vi "Get spec limits.vi"(0 "Zaber":T1={"Serial port handle"="", "Axis"="", "Controller #"=0, "Min position"=0.0, "Max position"=0.0, "Min velocity"=0.0, "Max velocity"=0.0, "Firmware"="", "Device ID"=0, "Variable event"=refnum, "Variable ref"=refnum, "Resolution, usteps/step"=0, "Serial port semaphore"=refnum, "Joystick buttons"={"MinDir"=1, "MaxDir"=2, "MedSpeed"=5, "HighSpeed"=6}} {"Joystick buttons"."HighSpeed" min=1 max=25 step=1; "Joystick buttons"."MedSpeed" min=1 max=25 step=1; "Joystick buttons"."MaxDir" min=1 max=25 step=1; "Joystick buttons"."MinDir" min=1 max=25 step=1}, 5 "error in":errorcluster) -> (14 "Zaber out":T1={"Serial port handle"="", "Axis"="", "Controller #"=0, "Min position"=0.0, "Max position"=0.0, "Min velocity"=0.0, "Max velocity"=0.0, "Firmware"="", "Device ID"=0, "Variable event"=refnum, "Variable ref"=refnum, "Resolution, usteps/step"=0, "Serial port semaphore"=refnum, "Joystick buttons"={"MinDir"=1, "MaxDir"=2, "MedSpeed"=5, "HighSpeed"=6}} {"Joystick buttons"."HighSpeed" min=1 max=25 step=1; "Joystick buttons"."MedSpeed" min=1 max=25 step=1; "Joystick buttons"."MaxDir" min=1 max=25 step=1; "Joystick buttons"."MinDir" min=1 max=25 step=1}, 15 "MAX velocity, mm/s":dbl, 16 "MIN velociry, mm/s":dbl, 17 "MIN position, mm":dbl, 19 "error out":errorcluster)   [LabVIEW 2018]
uses:
  Zaber.ctl
  GenericDataEvent/GenericEvent.ctl
  ZaberVariables.ctl
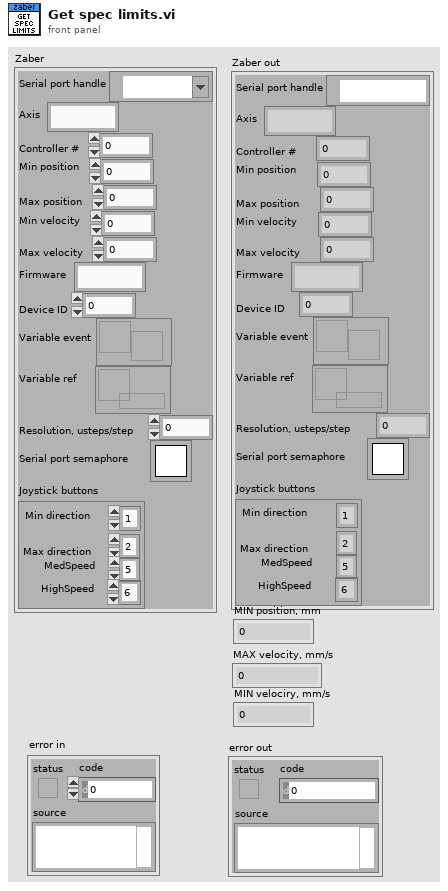
[diagram p1: front panel]
types:
  T1 = typedef "Zaber.ctl" = cluster{"Serial port handle":refnum<visa-resource-name>, "Axis":string, "Controller #":u8, "Min position":dbl, "Max position":dbl, "Min velocity":dbl, "Max velocity":dbl, "Firmware":string, "Device ID":i32, "Variable event":T2, "Variable ref":refnum<data-value>, "Resolution, usteps/step":i32, "Serial port semaphore":T3, "Joystick buttons":cluster{"MinDir":i32, "MaxDir":i32, "MedSpeed":i32, "HighSpeed":i32}}
  T2 = typedef "GenericEvent.ctl" = refnum<user-event>
  T3 = typedef "Semaphore RefNum" = refnum<k1>
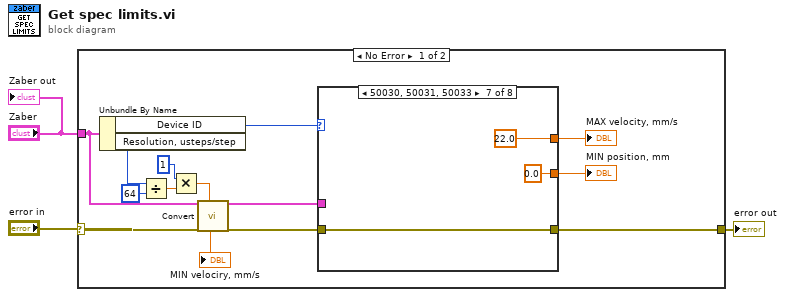
[diagram p0: block diagram]
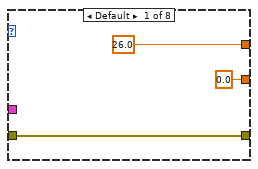
[diagram p2: hidden frame]
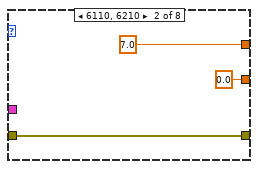
[diagram p3: hidden frame]
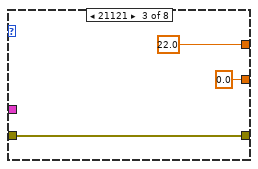
[diagram p4: hidden frame]
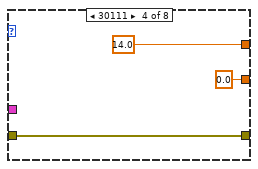
[diagram p5: hidden frame]
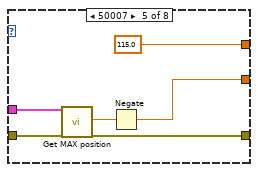
[diagram p6: hidden frame]
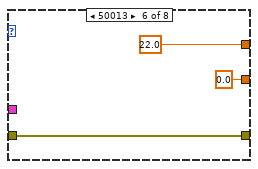
[diagram p7: hidden frame]
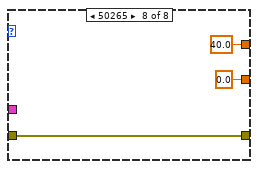
[diagram p8: hidden frame]
diagram:
  n1 = case shown="No Error" "error in" {
    selector: "error in" -> [w8 w45]
    tunnel: [w6 w45] -> w1
    tunnel: "Zaber" -> [w11 _]
    frame No Error {
      n2 = Unbundle By Name(w11) -> ("Device ID"=w17:i32, "Resolution, usteps/step"=w10:i32)
      n3 = Divide(x=w10, y=64) -> (x/y=w13:dbl)
      n4 = Multiply(x=1 ("Velocity, counts"), y=w13) -> (x*y=w15:dbl)
      n5 = call "Convert.vi"("Zaber"=w11, "error in"=w8, "Velocity, counts"=w15) -> ("Velocity, mm/s"=→"MIN velociry, mm/s":dbl, "Zaber out"=w4:T1, "error out"=w7:errorcluster)  [unwired: 8 in, 6 out]
      n6 = case shown="50030, 50031, 50033" w17 {
        tunnel: [26.0 ("upper limit") 7.0 ("upper limit") 22.0 ("upper limit") 14.0 ("upper limit") 115.0 ("upper limit") 22.0 ("upper limit") 22.0 ("upper limit") 40.0 ("upper limit")] -> w16
        tunnel: w7 -> [w18 w22 w25 w28 w34 w37 w39 w44]
        tunnel: [w18 w22 w25 w28 w33 w37 w39 w44] -> w6
        tunnel: [0.0 0.0 0.0 0.0 w31 0.0 0.0 0.0] -> w5
        tunnel: w4 -> [_ _ _ _ w30 _ _ _]
        frame Default {
        }
        frame 6110, 6210 {
        }
        frame 21121 {
        }
        frame 30111 {
        }
        frame 50007 {
          n7 = call "Get MAX position.vi"("Zaber"=w30, "error in"=w34) -> ("MAX position, mm"=w32:dbl, "error out"=w33:errorcluster)  [unwired: 14 in, 2 out]
          n8 = Negate(x=w32) -> (-x=w31:dbl)
        }
        frame 50013 {
        }
        frame 50030, 50031, 50033 {
        }
        frame 50265 {
        }
      }
      "MAX velocity, mm/s" <- w16
      "MIN position, mm" <- w5
    }
    frame Error {
    }
  }
  "error out" <- w1
  "Zaber out" <- "Zaber"
